vi "Set value by Variant.vi"(8 "error in (no error)":errorcluster, 10 "Variant":variant, 11 "Column in":refnum<class "Ctrl Refnum Column.lvclass">) -> (0 "error out":errorcluster, 3 "Column out":refnum<class "Ctrl Refnum Column.lvclass">)   [LabVIEW 2020, in "Basic Fields.lvlib" / "Ctrl Refnum Column.lvclass"]
uses:
  Ctrl Refnum Column.lvclass
  Ctrl Refnum Column.lvclass/Ctrl Refnum Column.ctl
  Basic Columns/Basic Columns/Column Class/Column Parent.lvclass
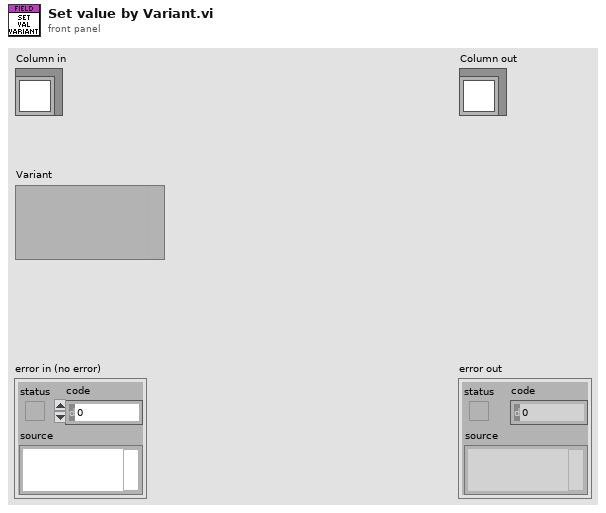
[diagram p1: front panel]
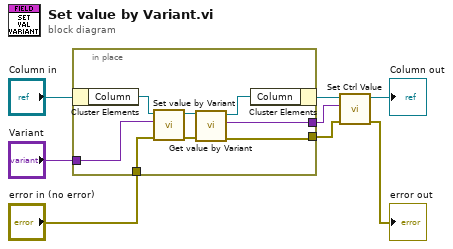
[diagram p0: block diagram]
diagram:
  n1 = in-place {
    in-place-border: "Variant" -> [w15]
    in-place-border: "error in (no error)" -> [w14]
    in-place-border: [w10] -> w4
    in-place-border: [w9] -> w1
    n2 = in-place-cluster #1("Column in") -> ("Column"=w16:refnum<class "Column Parent.lvclass">)
    n3 = call-dynamic "Set value by Variant.vi"("error in (no error)"=w14, "Variant"=w15, "Column in"=w16) -> ("error out"=w12:errorcluster, "Column out"=w13:refnum<class "Column Parent.lvclass">)  [unwired: 7 in]
    n4 = call-dynamic "Get value by Variant.vi"("error in (no error)"=w12, "Column Parent in"=w13) -> ("error out"=w10:errorcluster, "Variant"=w9:variant, "Column Parent out"=w11:refnum<class "Column Parent.lvclass">)  [unwired: 7 in]
    n5 = in-place-cluster #1("Column"=w11) -> (w5:refnum<class "Ctrl Refnum Column.lvclass">)
  }
  n6 = call-dynamic "Set Ctrl Value.vi"("error in (no error)"=w4, "Variant"=w1, "Ctrl Refnum Column in"=w5) -> ("error out"=→"error out":errorcluster, "Ctrl Refnum Column out"=→"Column out":refnum<class "Ctrl Refnum Column.lvclass">)  [unwired: 7 in]
